vi "Get Size From Tow Points.vi"(8 "error in (no error)":errorcluster caption="错误输入（无错误）", 11 "Point 输入":refnum<class "Point.lvclass"> caption="DNL_LabVIEW Object in") -> (0 "error out":errorcluster caption="错误输出")   [LabVIEW 2011, in "Point.lvclass"]
uses:
  Point.lvclass
  Size/Size.lvclass
panel:
  out "Size 输出":refnum<class "Size.lvclass">
  in  "Point 输入":refnum<class "Point.lvclass"> caption="DNL_LabVIEW Object in"
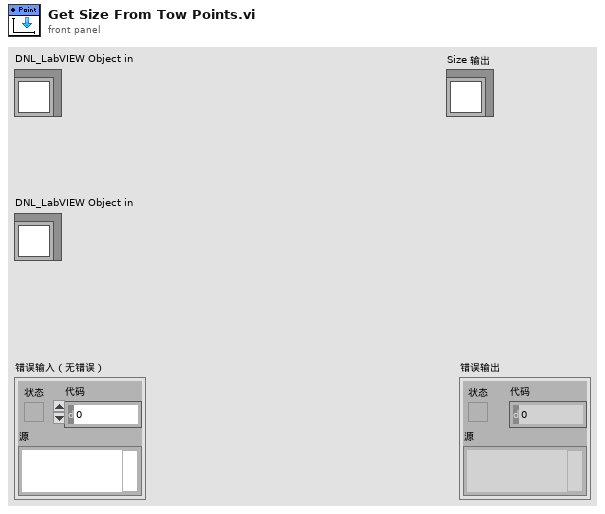
[diagram p1: front panel]
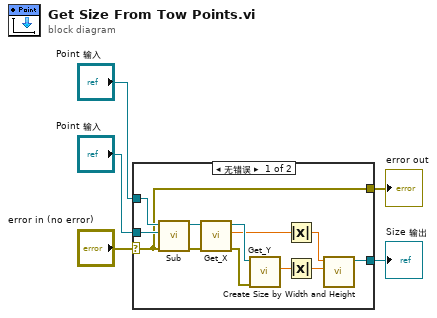
[diagram p0: block diagram]
diagram:
  n1 = case shown="无错误" "error in (no error)" {
    selector: "error in (no error)" -> [w15 w18]
    tunnel: [w15 w18] -> w4
    tunnel: "Point 输入" -> [w17 _]
    tunnel: "Point 输入" -> [w16 _]
    tunnel: [w6 _] -> w1
    frame No Error {
      n2 = call "Sub.vi"("error in (no error)"=w15, 10:"Point 输入"=w16, 11:"Point 输入"=w17) -> ("error out"=w13:errorcluster, "Point 输出"=w14:refnum<class "Point.lvclass">)  [unwired: 7 in]
      n3 = call "Get_X.vi"("error in (no error)"=w13, "Point输入"=w14) -> ("error out"=w11:errorcluster, "X"=w10:dbl, "Point输出"=w12:refnum<class "Point.lvclass">)  [unwired: 7 in]
      n4 = call "Get_Y.vi"("error in (no error)"=w11, "Point输入"=w12) -> ("Y"=w8:dbl)  [unwired: 7 in, 2 out]
      n5 = Absolute Value(x=w10) -> (abs(x)=w9:dbl)
      n6 = Absolute Value(x=w8) -> (abs(x)=w7:dbl)
      n7 = call "Create Size by Width and Height.vi"("Height"=w7, "Width"=w9) -> ("Size 输出"=w6:refnum<class "Size.lvclass">)  [unwired: 8 in, 1 out]
    }
    frame Error {
    }
  }
  "error out" <- w4
  "Size 输出" <- w1
